vi "Check Status.vi"(8 "error in":errorcluster, 11 "GOLPI ref. in":T1={"pipe handle"={"lv_proc.dll file path"=path "", "process instance handle"=[], "debug mode"=FALSE, "debug data"=[]}, "fast read timeout [ms]"=500, "fast read settle time [ms]"=10, "fast read to multiple [ms]"=1, "max elements per input line"=100, "slow read timeout [ms]"=5000, "stdin double format specifier"="", "max elements per stdout output column"=100}) -> (0 "error out":errorcluster, 2 "running?":bool, 3 "GOLPI ref. out":T1={"pipe handle"={"lv_proc.dll file path"=path "", "process instance handle"=[], "debug mode"=FALSE, "debug data"=[]}, "fast read timeout [ms]"=500, "fast read settle time [ms]"=10, "fast read to multiple [ms]"=1, "max elements per input line"=100, "slow read timeout [ms]"=5000, "stdin double format specifier"="", "max elements per stdout output column"=100})   [LabVIEW 2013, in "GOLPI library.lvlib"]
doc: "Check if GNU Octave is still running."
uses:
  GOLPI library.lvlib
  LV Process source distribution/LV Process library.lvlib
  GOLPI reference Type Def.ctl
  LV Process source distribution/Pipe Handle.ctl
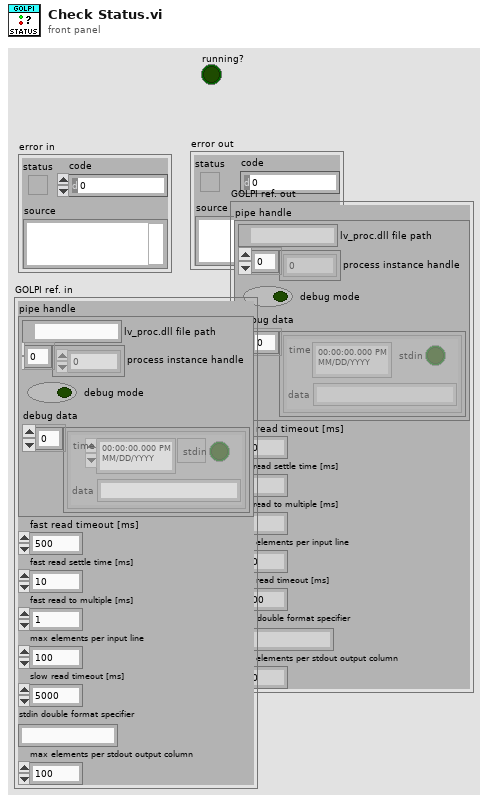
[diagram p1: front panel]
types:
  T1 = typedef "GOLPI library.lvlib/GOLPI reference Type Def.ctl" = cluster{"pipe handle":T2, "fast read timeout [ms]":u32, "fast read settle time [ms]":u32, "fast read to multiple [ms]":u32, "max elements per input line":u32, "slow read timeout [ms]":u32, "stdin double format specifier":string, "max elements per stdout output column":u32}
  T2 = typedef "LV Process library.lvlib/Pipe Handle.ctl" = cluster{"lv_proc.dll file path":path, "process instance handle":u32[], "debug mode":bool, "debug data":cluster{"time":timestamp, "stdin":bool, "data":string}[]}
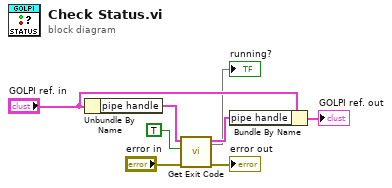
[diagram p0: block diagram]
diagram:
  n1 = Unbundle By Name("GOLPI ref. in") -> ("pipe handle"=w4:T2)
  n2 = call "Get Exit Code.vi"("error in"="error in", "ignore error if process running (T)"=TRUE ("ignore error if still active (T)"), "pipe in"=w4) -> ("error out"=→"error out":errorcluster, "pipe out"=w3:T2, 5:→"running?")  [unwired: 4 in, 2 out]
  n3 = Bundle By Name(cluster="GOLPI ref. in", "pipe handle"=w3) -> (→"GOLPI ref. out":T1)
